vi "New Test Name Dialog.vi"(8 "error in":errorcluster, 11 "M_Butt in":refnum<class "M_Butt.lvclass">) -> (0 "error out":errorcluster, 3 "M_Butt out":refnum<class "M_Butt.lvclass">)   [LabVIEW 2019, in "M_Butt.lvlib" / "M_Butt.lvclass"]
uses:
  Project/M_Butt.lvclass
  builds/Engine/Engine.lvlibp/Project/Engine.lvclass
  C:/Users/Public/Documents/Development/builds/Engine/Engine.lvlibp/Project/Engine.lvclass
panel:
  in  "Cancel":bool
  in  "OK":bool caption="OK2"
  in  "Enter New Test Name and press \"ok\"":string
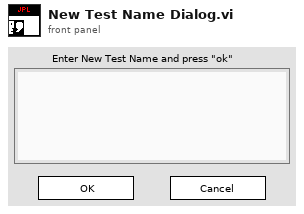
[diagram p1: front panel]
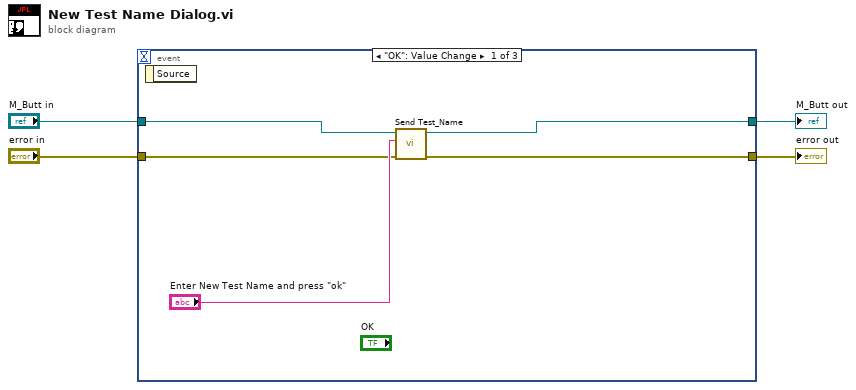
[diagram p0: block diagram]
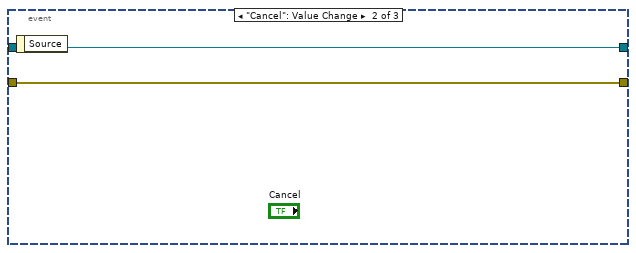
[diagram p2: hidden frame]
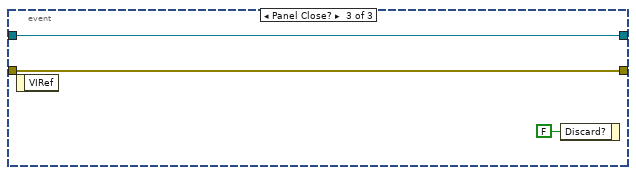
[diagram p3: hidden frame]
diagram:
  n1 = event shown="[0] \"OK\": Value Change" {
    selector: _ -> [_ _ _]
    dyn-events: _ -> [_ _ _]
    timeout: _ -> [_ _ _]
    tunnel: "M_Butt in" -> [w9 w11 w14]
    tunnel: [w6 w11 w14] -> w3
    tunnel: "error in" -> [w7 w10 w13]
    tunnel: [w5 w10 w13] -> w1
    event "OK": Value Change {
      n2 = event-data() -> ()  [unwired: 1 in, 1 out]
      n3 = call "Send Test_Name.vi"("error in"=w7, "Test Name"="Enter New Test Name and press \"ok\"", "Engine in"=w9) -> ("error out"=w5:errorcluster, "Engine out"=w6:refnum<class "M_Butt.lvclass">)  [unwired: 7 in]
    }
    event "Cancel": Value Change {
      n4 = event-data() -> ()  [unwired: 1 in, 1 out]
    }
    event Panel Close? {
      n5 = event-data() -> ()  [unwired: 1 in, 1 out]
      n6 = event-data("Discard?"=FALSE) -> ()  [unwired: 1 in, 1 out]
    }
  }
  "error out" <- w1
  "M_Butt out" <- w3
